vi "Class Icon Name.vi"(8 "Error In":errorcluster, 11 "Value":variant) -> (0 "Error Out":errorcluster, 3 "String":string)   [LabVIEW 2018, in "Scripts.lvlib"]
uses:
  Scripts.lvlib
  <vilib>/Utility/Data Type/NI_Data Type.lvlib
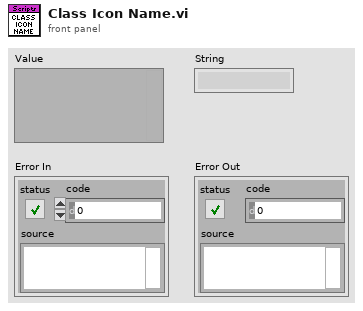
[diagram p1: front panel]
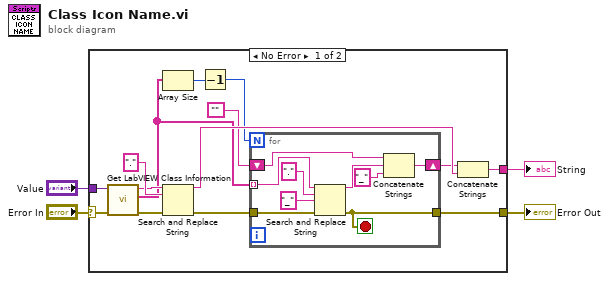
[diagram p0: block diagram]
diagram:
  n1 = case shown="No Error" "Error In" {
    selector: "Error In" -> [w5 w28]
    tunnel: [w16 _] -> w4
    tunnel: [w8 w28] -> w3
    tunnel: "Value" -> [w6 _]
    frame No Error {
      n2 = call <vilib>:"Get LabVIEW Class Information.vi"("error in (no error)"=w5, "Variant"=w6) -> ("error out"=w14:errorcluster, "Qualified LabVIEW Class Name"=w9:string[], "LabVIEW Class File Name"=w12:string)  [unwired: 7 in]
      n3 = Array Size(array=w9) -> (size(s)=w10:i32)
      n4 = Search and Replace String(input string=w12, search string=".", error in=w14) -> (result string=w18:string, error out=w15:errorcluster)  [unwired: 5 in, 2 out]
      n5 = Decrement(x=w10) -> (x-1=w11:i32)
      n6 = for {
        N: w11 -> [_]
        tunnel: w9 -> [w25] mode=indexing
        shift-right: [w26] -> w17
        shift-left: "" -> [w27]
        tunnel: w15 -> [w22]
        tunnel: [w21] -> w8
        stop <- w21 stop-if-true
        n7 = Search and Replace String(input string=w25, search string=".", replace string="_" ("replace string (\"\")"), error in=w22) -> (result string=w20:string, error out=w21:errorcluster)  [unwired: 4 in, 2 out]
        n8 = Concatenate Strings(w27, w20, "_" ("string")) -> (w26:string)
      }
      n9 = Concatenate Strings(w17, w18) -> (w16:string)
    }
    frame Error {
    }
  }
  "String" <- w4
  "Error Out" <- w3
